vi "Gasteiler KommVI.vi"() -> (0 "error IO":errorcluster, 3 "Verfügbare Gase 2":string[][](table))   [LabVIEW 2020, in "Linearisierung v2.lvlib" / "Gasteiler.lvlib"]
uses:
  Gasteiler.lvlib
  Aktion Gasteiler KommVI.ctl
  AK-Komm Gasteiler/Aktionen AK Komm.ctl
  AK-Komm Gasteiler/Alter Gasteiler/Aktionen AK Komm_ALT.ctl
  Horiba/Aktion Befehl.ctl
  Aktionen FGV Gasteiler Daten.ctl
  Aktion unterbrechen.ctl
  Aktion FGV Stoerungen sammeln und auswerten.ctl
  Daten abholen.ctl
  AK-Komm Gasteiler/AK Komm Gasteiler.lvlib
  AK-Komm Gasteiler/Alter Gasteiler/Alter Gasteiler.lvlib
  Horiba/Horiba GDC.lvlib
  EPA1065-307/Linearity verification 1065-307.lvlib
  Linearisierung v2.lvlib
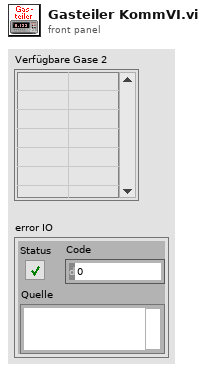
[diagram p1: front panel]
types:
  T1 = typedef "Linearisierung v2.lvlib/Gasteiler.lvlib/Aktion unterbrechen.ctl" = enum16{"Betrieb", "Unterbrechen", "Warten"}
  T2 = typedef "Linearisierung v2.lvlib/Gasteiler.lvlib/Aktionen FGV Gasteiler Daten.ctl" = enum16{"lesen", "Gasteiler Daten", "Seriellen Param.", "MB-Endwert", "laden", "speichern", "Anforderung", "TCP", "Aufzeichnung Start"}
  T3 = typedef "Linearisierung v2.lvlib/Gasteiler.lvlib/Horiba GDC.lvlib/Aktion Befehl.ctl" = enum16{"lesen", "initialisieren", "Beenden", "Standby", "GD/CC", "Info", "Flow", "Alarm", "GD parameter", "GD point", "Durchfluss", "Spuelen1", "Spuelen1 On", "Spuelen1Off", "Spuelen2", "Ventil-Abfrage", "Reset"}
  T4 = typedef "Linearisierung v2.lvlib/Gasteiler.lvlib/AK Komm Gasteiler.lvlib/Alter Gasteiler.lvlib/Aktionen AK Komm_ALT.ctl" = enum16{"lesen", "initialisieren", "beenden", "SRES", "STBY", "SREM", "SMAN", "SLIN", "SLCH", "SLST", "SSPL", "AGAT", "ALST", "ASTZ", "ASTF", "AGAK", "EGAK"}
  T5 = typedef "Linearisierung v2.lvlib/Gasteiler.lvlib/AK Komm Gasteiler.lvlib/Aktionen AK Komm.ctl" = enum16{"lesen", "initialisieren", "beenden", "Status", "SMAN", "SREM", "STBY", "ASTF", "ASTZ", "SLST", "AGAT", "EGAK", "AGAK", "AKAK", "ADRU", "SKOP", "SVSA", "SVSZ", "SONO", "SAIR", "SNOX", "ANOX", "SSPL", "SRUC", "SLIN", "ALST", "ETYP", "SVIO", "LCYL", "CCYL", "DCYL", "SCYL", "GCYL", "DRGV", "DRDC"}
  T6 = typedef "Linearisierung v2.lvlib/Gasteiler.lvlib/Aktion Gasteiler KommVI.ctl" = enum16{"Init", "verbinden", "komm", "beenden"}
  T7 = typedef "Linearisierung v2.lvlib/Daten abholen.ctl" = enum16{"Initialisieren", "Punkt aufschalten", "Warten", "Daten abholen", "Fertig", "Beenden", "Spülen", "Abbrechen"}
  T8 = typedef "Linearisierung v2.lvlib/Aktion FGV Stoerungen sammeln und auswerten.ctl" = enum16{"init", "lesen", "error", "prüfen", "reset error", "abbrechen", "fortsetzen", "neustart", "Bedientasten reset"}
  T9 = typedef "Linearisierung v2.lvlib/Gasteiler.lvlib/Gasteiler Daten.ctl" = cluster{"Gasteiler":T10, "Gasteiler Stufen":T11, "Gasteiler Type":T12, "Konfig Gasteiler":T13, "Gasteiler Span Eingänge":u16}
  T10 = typedef "String - Eingabefeld.ctl" = string
  T11 = typedef "Linearisierung v2.lvlib/Gasteiler.lvlib/Gasteiler Stufen.ctl" = u16
  T12 = typedef "Linearisierung v2.lvlib/GasteilerType.ctl" = u16
  T13 = typedef "System Einstellungen V2.lvlib/Gasteiler Auswahl.ctl" = u16
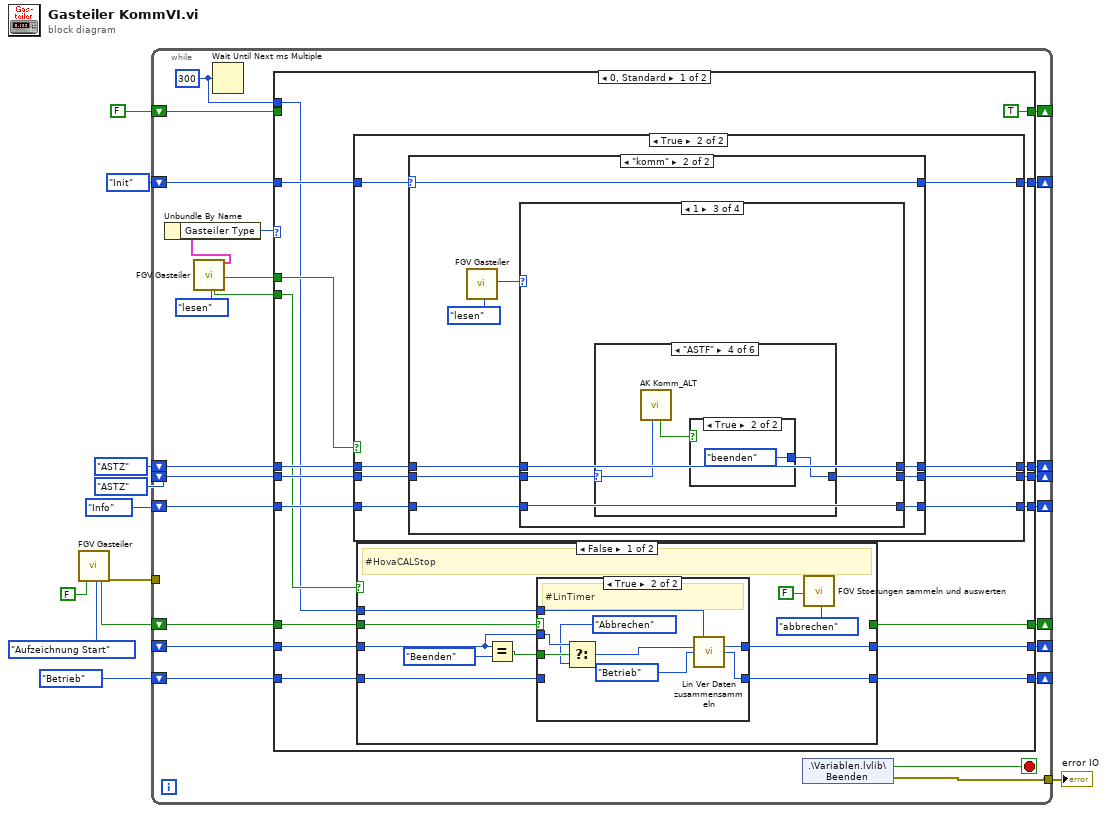
[diagram p0: block diagram]
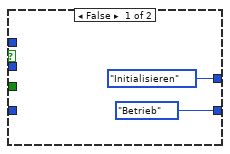
[diagram p2: hidden frame]
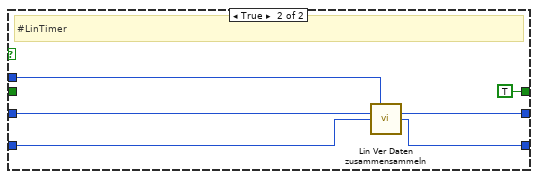
[diagram p3: hidden frame]
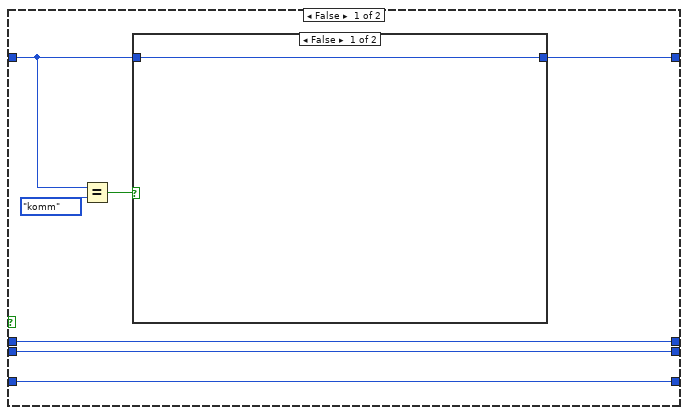
[diagram p4: hidden frame]
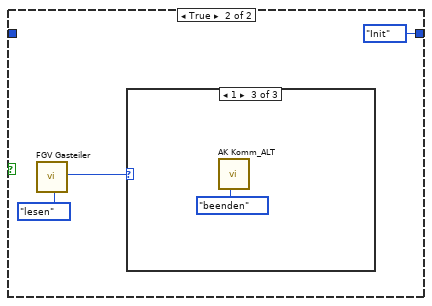
[diagram p5: hidden frame]
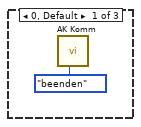
[diagram p6: hidden frame]
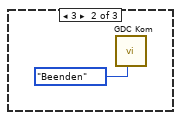
[diagram p7: hidden frame]
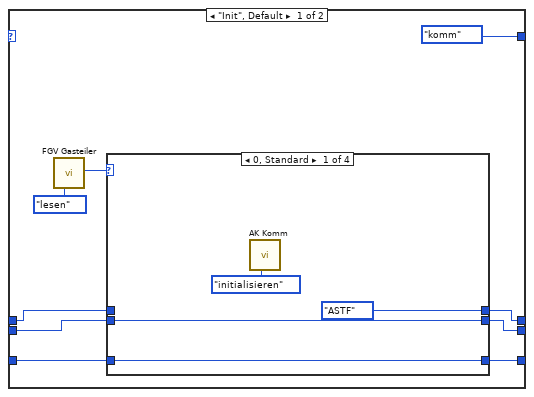
[diagram p8: hidden frame]
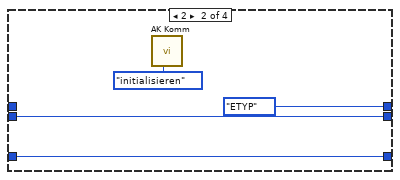
[diagram p9: hidden frame]
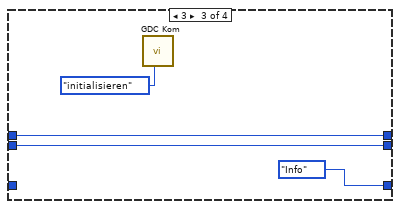
[diagram p10: hidden frame]
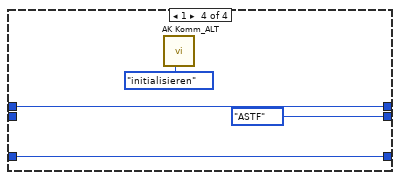
[diagram p11: hidden frame]
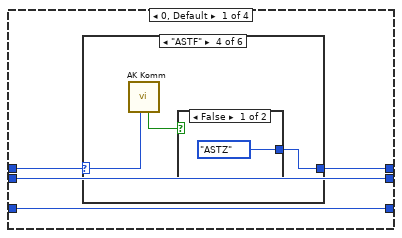
[diagram p12: hidden frame]
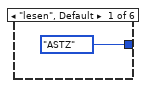
[diagram p13: hidden frame]
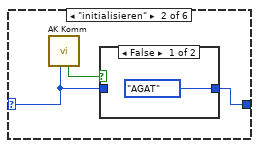
[diagram p14: hidden frame]
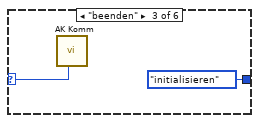
[diagram p16: hidden frame]
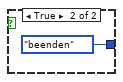
[diagram p17: hidden frame]
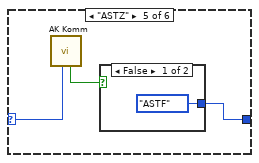
[diagram p18: hidden frame]
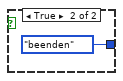
[diagram p19: hidden frame]
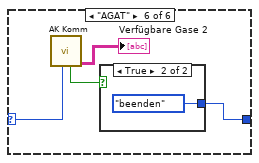
[diagram p20: hidden frame]
diagram:
  n1 = call "FGV Gasteiler.vi"("Aufzeichnung Start"=FALSE, "Aktionen"=Aktionen_FGV_Gasteiler_Daten."Aufzeichnung Start") -> ("Aufzeichnung Start"=w3:bool, "error out"=w4:errorcluster)  [unwired: 10 in, 6 out]
  n2 = while {
    shift-right: [w33] -> _
    shift-left: Aktionen_AK_Komm_ALT."ASTZ" ("Aktionen_ALT") -> [w31]
    shift-right: [w34] -> _
    shift-left: Aktionen_AK_Komm."ASTZ" ("Aktionen") -> [w32]
    shift-right: [w29] -> _
    shift-left: Aktion_Gasteiler_KommVI."Init" ("Aktion") -> [w30]
    tunnel: [w26] -> w8
    shift-right: [w25] -> _
    shift-left: Aktion_Befehl."Info" ("Befehl") -> [w24]
    shift-right: [w23] -> _
    shift-left: _ -> [w22]
    tunnel: w4 -> [_]
    shift-right: [w19] -> _
    shift-left: w3 -> [w20]
    shift-right: [w15] -> _
    shift-left: FALSE ("Aufzeichnung Start") -> [w16]
    shift-right: [w13] -> _
    shift-left: Aktion_unterbrechen."Betrieb" ("Aktion Unterbrechen") -> [w14]
    stop <- w35 stop-if-true
    w12 = u32 300 ("Vielfache von ms")
    n3 = call "FGV Gasteiler.vi"("Aktionen"=Aktionen_FGV_Gasteiler_Daten."lesen") -> ("Aufzeichnung Start"=w21:bool, "Gasteiler Daten"=w18:T9, "Anforderung"=w27:bool)  [unwired: 11 in, 5 out]
    n4 = Unbundle By Name(w18) -> ("Gasteiler Type"=w17:T12)
    n5 = Wait Until Next ms Multiple(millisecond multiple=w12) -> ()  [unwired: 1 out]
    n6 = case shown="0, Standard" w17 {
      tunnel: [w53 Aktionen_AK_Komm."ASTZ" ("Aktionen")] -> w34
      tunnel: [w52 Aktionen_AK_Komm_ALT."ASTZ" ("Aktionen_ALT")] -> w33
      tunnel: w32 -> [w51 _]
      tunnel: w31 -> [w50 _]
      tunnel: w30 -> [w49 _]
      tunnel: [w48 Aktion_Gasteiler_KommVI."Init" ("Aktion")] -> w29
      tunnel: w27 -> [w47 _]
      tunnel: [w46 Aktion_Befehl."Info" ("Befehl")] -> w25
      tunnel: w24 -> [w45 _]
      tunnel: [w44 w264] -> w23
      tunnel: w22 -> [w43 w264]
      tunnel: w21 -> [w42 _]
      tunnel: w20 -> [w41 _]
      tunnel: [w40 FALSE ("Aufzeichnung Start")] -> w19
      tunnel: w16 -> [_ w263]
      tunnel: [TRUE w262] -> w15
      tunnel: w14 -> [w38 w261]
      tunnel: [w37 w261] -> w13
      tunnel: w12 -> [w36 _]
      frame 0, Default {
        n7 = case shown="True" w47 {
          tunnel: [w86 w101] -> w53
          tunnel: [w85 w100] -> w52
          tunnel: w51 -> [w86 w99]
          tunnel: w50 -> [w85 w98]
          tunnel: w49 -> [w82 w97]
          tunnel: [w81 w96] -> w48
          tunnel: [w80 w95] -> w46
          tunnel: w45 -> [w80 w94]
          frame False {
            n8 = Equal?(x=w82, y=Aktion_Gasteiler_KommVI."komm") -> (x = y?=w83:bool)
            n9 = case shown="False" w83 {
              tunnel: [w87 Aktion_Gasteiler_KommVI."Init" ("Aktion")] -> w81
              tunnel: w82 -> [w87 _]
              frame False {
              }
              frame True {
                n10 = call "FGV Gasteiler.vi"("Aktionen"=Aktionen_FGV_Gasteiler_Daten."lesen") -> ("Gasteiler Type"=w89:T12)  [unwired: 11 in, 7 out]
                n11 = case shown="1" w89 {
                  frame 0, Default {
                    n12 = call "AK Komm.vi"("Aktionen"=Aktionen_AK_Komm."beenden") -> ()  [unwired: 4 in, 7 out]
                  }
                  frame 3 {
                    n13 = call "GDC Kom.vi"("Befehl"=Aktion_Befehl."Beenden") -> ()  [unwired: 4 in, 7 out]
                  }
                  frame 1 {
                    n14 = call "AK Komm_ALT.vi"("Aktionen_ALT"=Aktionen_AK_Komm_ALT."beenden") -> ()  [unwired: 6 in, 5 out]
                  }
                }
              }
            }
          }
          frame True {
            n15 = case shown="\"komm\"" w97 {
              selector: w97 -> [_ w129]
              tunnel: [w105 w133] -> w101
              tunnel: [w104 w132] -> w100
              tunnel: w99 -> [w107 w131]
              tunnel: w98 -> [w106 w130]
              tunnel: [Aktion_Gasteiler_KommVI."komm" ("Aktion") w129] -> w96
              tunnel: [w103 w128] -> w95
              tunnel: w94 -> [w102 w127]
              frame "Init", Default {
                n16 = call "FGV Gasteiler.vi"("Aktionen"=Aktionen_FGV_Gasteiler_Daten."lesen") -> ("Gasteiler Type"=w108:T12)  [unwired: 11 in, 7 out]
                n17 = case shown="0, Standard" w108 {
                  tunnel: w107 -> [_ _ w121 w125]
                  tunnel: [Aktionen_AK_Komm."ASTF" ("Aktionen") Aktionen_AK_Komm."ETYP" ("Aktionen") w121 w125] -> w105
                  tunnel: w106 -> [w113 w117 w119 _]
                  tunnel: [w113 w117 w119 Aktionen_AK_Komm_ALT."ASTF" ("Aktionen_ALT")] -> w104
                  tunnel: [w111 w115 Aktion_Befehl."Info" ("Befehl") w123] -> w103
                  tunnel: w102 -> [w111 w115 _ w123]
                  frame 0, Default {
                    n18 = call "AK Komm.vi"("Aktionen"=Aktionen_AK_Komm."initialisieren") -> ()  [unwired: 4 in, 7 out]
                  }
                  frame 2 {
                    n19 = call "AK Komm.vi"("Aktionen"=Aktionen_AK_Komm."initialisieren") -> ()  [unwired: 4 in, 7 out]
                  }
                  frame 3 {
                    n20 = call "GDC Kom.vi"("Befehl"=Aktion_Befehl."initialisieren") -> ()  [unwired: 4 in, 7 out]
                  }
                  frame 1 {
                    n21 = call "AK Komm_ALT.vi"("Aktionen_ALT"=Aktionen_AK_Komm_ALT."initialisieren") -> ()  [unwired: 6 in, 5 out]
                  }
                }
              }
              frame "komm" {
                n22 = call "FGV Gasteiler.vi"("Aktionen"=Aktionen_FGV_Gasteiler_Daten."lesen") -> ("Gasteiler Type"=w134:T12)  [unwired: 11 in, 7 out]
                n23 = case shown="1" w134 {
                  tunnel: w131 -> [w139 w164 w212 w236]
                  tunnel: [w138 w167 w212 w236] -> w133
                  tunnel: w130 -> [w137 w166 w211 w237]
                  tunnel: [w137 w166 w210 w237] -> w132
                  tunnel: [w136 w165 w209 w239] -> w128
                  tunnel: w127 -> [w136 w165 w209 w238]
                  frame 0, Default {
                    n24 = case shown="\"ASTF\"" w139 {
                      selector: w139 -> [_ w141 w147 w149 w155 w161]
                      tunnel: [Aktionen_AK_Komm."ASTZ" ("Aktionen") w142 Aktionen_AK_Komm."initialisieren" ("Aktionen") w148 w153 w159] -> w138
                      frame "lesen", Default {
                      }
                      frame "initialisieren" {
                        n25 = call "AK Komm.vi"("Aktionen"=w141) -> ("Störung Kommunikation"=w143:bool)  [unwired: 4 in, 6 out]
                        n26 = case shown="False" w143 {
                          tunnel: [Aktionen_AK_Komm."AGAT" ("Aktionen") w145] -> w142
                          tunnel: w141 -> [_ w145]
                          frame False {
                          }
                          frame True {
                          }
                        }
                      }
                      frame "beenden" {
                        n27 = call "AK Komm.vi"("Aktionen"=w147) -> ()  [unwired: 4 in, 7 out]
                      }
                      frame "ASTF" {
                        n28 = call "AK Komm.vi"("Aktionen"=w149) -> ("Störung Kommunikation"=w150:bool)  [unwired: 4 in, 6 out]
                        n29 = case shown="False" w150 {
                          tunnel: [Aktionen_AK_Komm."ASTZ" ("Aktionen") Aktionen_AK_Komm."beenden" ("Aktionen")] -> w148
                          frame False {
                          }
                          frame True {
                          }
                        }
                      }
                      frame "ASTZ" {
                        n30 = call "AK Komm.vi"("Aktionen"=w155) -> ("Störung Kommunikation"=w154:bool)  [unwired: 4 in, 6 out]
                        n31 = case shown="False" w154 {
                          tunnel: [Aktionen_AK_Komm."ASTF" ("Aktionen") Aktionen_AK_Komm."beenden" ("Aktionen")] -> w153
                          frame False {
                          }
                          frame True {
                          }
                        }
                      }
                      frame "AGAT" {
                        n32 = call "AK Komm.vi"("Aktionen"=w161) -> ("Verfügbare Gase"=→"Verfügbare Gase 2":string[][], "Störung Kommunikation"=w160:bool)  [unwired: 4 in, 5 out]
                        n33 = case shown="True" w160 {
                          tunnel: [Aktionen_AK_Komm."ASTZ" ("Aktionen") Aktionen_AK_Komm."beenden" ("Aktionen")] -> w159
                          frame False {
                          }
                          frame True {
                          }
                        }
                      }
                    }
                  }
                  frame 2 {
                    n34 = case shown="\"ETYP\"" w164 {
                      selector: w164 -> [_ w169 w175 w177 w183 w192 w200 w206]
                      tunnel: [Aktionen_AK_Komm."ASTZ" ("Aktionen") w170 Aktionen_AK_Komm."initialisieren" ("Aktionen") w176 w182 w190 w198 w204] -> w167
                      frame "lesen", Default {
                      }
                      frame "initialisieren" {
                        n35 = call "AK Komm.vi"("Aktionen"=w169) -> ("Störung Kommunikation"=w171:bool)  [unwired: 4 in, 6 out]
                        n36 = case shown="False" w171 {
                          tunnel: [Aktionen_AK_Komm."AGAT" ("Aktionen") w173] -> w170
                          tunnel: w169 -> [_ w173]
                          frame False {
                          }
                          frame True {
                          }
                        }
                      }
                      frame "beenden" {
                        n37 = call "AK Komm.vi"("Aktionen"=w175) -> ()  [unwired: 4 in, 7 out]
                      }
                      frame "ASTF" {
                        n38 = call "AK Komm.vi"("Aktionen"=w177) -> ("Störung Kommunikation"=w178:bool)  [unwired: 4 in, 6 out]
                        n39 = case shown="True" w178 {
                          tunnel: [Aktionen_AK_Komm."ASTZ" ("Aktionen") Aktionen_AK_Komm."beenden" ("Aktionen")] -> w176
                          frame False {
                          }
                          frame True {
                          }
                        }
                      }
                      frame "ETYP" {
                        n40 = call "AK Komm.vi"("Aktionen"=w183, "Daten"=string[] ["4"]) -> ("Störung Kommunikation"=w184:bool)  [unwired: 3 in, 6 out]
                        n41 = case shown="True" w184 {
                          tunnel: [Aktionen_AK_Komm."ASTF" ("Aktionen") Aktionen_AK_Komm."beenden" ("Aktionen")] -> w182
                          frame False {
                          }
                          frame True {
                          }
                        }
                      }
                      frame "ASTZ" {
                        n42 = call "AK Komm.vi"("Aktionen"=w192) -> ("Störung Kommunikation"=w191:bool, "Betriebsart"=w189:string)  [unwired: 4 in, 5 out]
                        n43 = Not Equal?(x=w189, y="SREM") -> (x != y?=w187:bool)
                        n44 = case shown="False" w187 {
                          tunnel: w191 -> [w194 _]
                          tunnel: [w193 Aktionen_AK_Komm."SREM" ("Aktionen")] -> w190
                          frame False {
                            n45 = case shown="False" w194 {
                              tunnel: [Aktionen_AK_Komm."ASTF" ("Aktionen") Aktionen_AK_Komm."beenden" ("Aktionen")] -> w193
                              frame False {
                              }
                              frame True {
                              }
                            }
                          }
                          frame True {
                          }
                        }
                      }
                      frame "SREM" {
                        n46 = call "AK Komm.vi"("Aktionen"=w200) -> ("Störung Kommunikation"=w199:bool)  [unwired: 4 in, 6 out]
                        n47 = case shown="False" w199 {
                          tunnel: [Aktionen_AK_Komm."ETYP" ("Aktionen") Aktionen_AK_Komm."beenden" ("Aktionen")] -> w198
                          frame False {
                          }
                          frame True {
                          }
                        }
                      }
                      frame "AGAT" {
                        n48 = call "AK Komm.vi"("Aktionen"=w206) -> ("Verfügbare Gase"=w203:string[][], "Störung Kommunikation"=w205:bool)  [unwired: 4 in, 5 out]
                        n49 = case shown="True" w205 {
                          tunnel: [Aktionen_AK_Komm."ASTZ" ("Aktionen") Aktionen_AK_Komm."beenden" ("Aktionen")] -> w204
                          frame False {
                          }
                          frame True {
                          }
                        }
                        n50 = local write "Verfügbare Gase 2"(w203) -> ()
                      }
                    }
                  }
                  frame 1 {
                    n51 = case shown="\"ASTF\"" w211 {
                      selector: w211 -> [_ w214 w220 w222 w228 w233]
                      tunnel: [Aktionen_AK_Komm_ALT."ASTZ" ("Aktionen_ALT") w215 Aktionen_AK_Komm_ALT."initialisieren" ("Aktionen_ALT") w221 w226 w231] -> w210
                      frame "lesen", Default {
                      }
                      frame "initialisieren" {
                        n52 = call "AK Komm_ALT.vi"("Aktionen_ALT"=w214) -> ("Störung Kommunikation"=w216:bool)  [unwired: 6 in, 4 out]
                        n53 = case shown="True" w216 {
                          tunnel: [Aktionen_AK_Komm_ALT."ASTZ" ("Aktionen_ALT") w218] -> w215
                          tunnel: w214 -> [_ w218]
                          frame False {
                          }
                          frame True {
                          }
                        }
                      }
                      frame "beenden" {
                        n54 = call "AK Komm_ALT.vi"("Aktionen_ALT"=w220) -> ()  [unwired: 6 in, 5 out]
                      }
                      frame "ASTF" {
                        n55 = call "AK Komm_ALT.vi"("Aktionen_ALT"=w222) -> ("Störung Kommunikation"=w223:bool)  [unwired: 6 in, 4 out]
                        n56 = case shown="True" w223 {
                          tunnel: [Aktionen_AK_Komm_ALT."ASTZ" ("Aktionen_ALT") Aktionen_AK_Komm_ALT."beenden" ("Aktionen_ALT")] -> w221
                          frame False {
                          }
                          frame True {
                          }
                        }
                      }
                      frame "ASTZ" {
                        n57 = call "AK Komm_ALT.vi"("Aktionen_ALT"=w228) -> ("Störung Kommunikation"=w227:bool)  [unwired: 6 in, 4 out]
                        n58 = case shown="False" w227 {
                          tunnel: [Aktionen_AK_Komm_ALT."ASTF" ("Aktionen_ALT") Aktionen_AK_Komm_ALT."beenden" ("Aktionen_ALT")] -> w226
                          frame False {
                          }
                          frame True {
                          }
                        }
                      }
                      frame "AGAT" {
                        n59 = call "AK Komm_ALT.vi"("Aktionen_ALT"=w233) -> ("Störung Kommunikation"=w232:bool)  [unwired: 6 in, 4 out]
                        n60 = case shown="False" w232 {
                          tunnel: [Aktionen_AK_Komm_ALT."ASTZ" ("Aktionen_ALT") Aktionen_AK_Komm_ALT."beenden" ("Aktionen_ALT")] -> w231
                          frame False {
                          }
                          frame True {
                          }
                        }
                      }
                    }
                  }
                  frame 3 {
                    n61 = case shown="\"Info\"" w238 {
                      tunnel: [Aktion_Befehl."Info" ("Befehl") w243 w247 w252 w258] -> w239
                      frame "lesen", Default {
                      }
                      frame "initialisieren" {
                        n62 = call "GDC Kom.vi"("Befehl"=Aktion_Befehl."initialisieren") -> ("Fehler"=w242:bool)  [unwired: 4 in, 6 out]
                        n63 = case shown="False" w242 {
                          tunnel: [Aktion_Befehl."Info" ("Befehl") Aktion_Befehl."initialisieren" ("Befehl")] -> w243
                          frame False {
                          }
                          frame True {
                          }
                        }
                      }
                      frame "Alarm" {
                        n64 = call "GDC Kom.vi"("Befehl"=Aktion_Befehl."Alarm") -> ("Fehler"=w246:bool)  [unwired: 4 in, 6 out]
                        n65 = case shown="False" w246 {
                          tunnel: [Aktion_Befehl."Flow" ("Befehl") Aktion_Befehl."initialisieren" ("Befehl")] -> w247
                          frame False {
                          }
                          frame True {
                          }
                        }
                      }
                      frame "Flow" {
                        n66 = call "GDC Kom.vi"("Befehl"=Aktion_Befehl."Flow") -> ("Fehler"=w251:bool)  [unwired: 4 in, 6 out]
                        n67 = case shown="False" w251 {
                          tunnel: [Aktion_Befehl."Info" ("Befehl") Aktion_Befehl."initialisieren" ("Befehl")] -> w252
                          frame False {
                          }
                          frame True {
                          }
                        }
                      }
                      frame "Info" {
                        n68 = call "GDC Kom.vi"("Befehl"=Aktion_Befehl."Info") -> ("Fehler"=w257:bool)  [unwired: 4 in, 6 out]
                        n69 = case shown="False" w257 {
                          tunnel: [Aktion_Befehl."Alarm" ("Befehl") Aktion_Befehl."initialisieren" ("Befehl")] -> w258
                          frame False {
                          }
                          frame True {
                          }
                        }
                      }
                    }
                  }
                }
              }
            }
          }
        }
        n70 = case shown="False" w42 {
          tunnel: w43 -> [w55 w79]
          tunnel: [w63 w78] -> w44
          tunnel: w41 -> [w62 _]
          tunnel: [_ TRUE ("Aufzeichnung Start")] -> w40
          tunnel: w38 -> [w58 w76]
          tunnel: [w59 w75] -> w37
          tunnel: w36 -> [w54 w74]
          frame False {
            # "#HovaCALStop"
            n71 = Equal?(x=w55, y=Daten_abholen."Beenden") -> (x = y?=w56:bool)
            n72 = case shown="True" w62 {
              tunnel: [Daten_abholen."Initialisieren" ("Aktionen Daten abholen") w73] -> w63
              tunnel: [Aktion_unterbrechen."Betrieb" ("Aktion Unterbrechen") w72] -> w59
              tunnel: w58 -> [_ _]
              tunnel: w56 -> [_ w70]
              tunnel: w55 -> [_ w69]
              tunnel: w54 -> [_ w66]
              frame False {
              }
              frame True {
                # "#LinTimer"
                n73 = Select(t=w69, s=w70, f=Daten_abholen."Abbrechen" ("Aktionen Daten abholen")) -> (s? t:f=w68:T7)
                n74 = call "Lin Ver Daten zusammensammeln.vi"("KommLoopTimer"=w66, "Aktionen Daten abholen"=w68, "Aktion Unterbrechen"=Aktion_unterbrechen."Betrieb") -> ("Aktionen Daten abholen"=w73:T7, "Aktion Unterbrechen"=w72:T1)  [unwired: 8 in, 3 out]
              }
            }
            n75 = call "FGV Stoerungen sammeln und auswerten.vi"("Abbrechen"=FALSE, "Aktion"=Aktion_FGV_Stoerungen_sammeln_und_auswerten."abbrechen") -> ()  [unwired: 11 in, 7 out]
          }
          frame True {
            # "#LinTimer"
            n76 = call "Lin Ver Daten zusammensammeln.vi"("KommLoopTimer"=w74, "Aktionen Daten abholen"=w79, "Aktion Unterbrechen"=w76) -> ("Aktionen Daten abholen"=w78:T7, "Aktion Unterbrechen"=w75:T1)  [unwired: 8 in, 3 out]
          }
        }
      }
      frame 4 {
        n77 = case shown="True" w263 {
          selector: w263 -> [w270 _]
          tunnel: [w270 FALSE] -> w262
          frame False {
          }
          frame True {
            # "Alle anderen deaktivieren"
            n78 = call "GDC Kom.vi"("Befehl"=Aktion_Befehl."Beenden") -> ()  [unwired: 4 in, 7 out]
            n79 = call "AK Komm_ALT.vi"("Aktionen_ALT"=Aktionen_AK_Komm_ALT."beenden") -> ()  [unwired: 6 in, 5 out]
            n80 = call "AK Komm.vi"("Aktionen"=Aktionen_AK_Komm."beenden") -> ()  [unwired: 4 in, 7 out]
          }
        }
      }
    }
    n81 = shared-variable ".\\Variablen.lvlib\\Beenden"() -> (w35:bool, error out=w26:errorcluster)  [unwired: 1 out]
  }
  "error IO" <- w8
